vi "drive_straight4.vi"(4 "YawRate_Meas":dbl, 6 "YawTgt":dbl, 7 "Output Power Limit":dbl=0.35 format="%#_13g", 8 "YawMeas":dbl, 9 "Init":bool, 10 "DistanceTgt":dbl, 11 "EncoderVal":T1) -> (2 "Done":bool, 3 "MotorCmdOut":cluster{"left":dbl, "right":dbl})   [LabVIEW 2015]
panel:
  in  "Ernie DC_Yaw_Kp":dbl=0.03
  out "Drive":cluster{dbl, "Output Power Limit":dbl}(graph)
  out "DiffCtrl":cluster{dbl, "Output Power Limit":dbl}(graph)
  out "Yaw Graph":dbl(graph)
  in  "Position Error Limit Negative":dbl=-4.0
  in  "Position Error Limit Positive":dbl
  in  "DC_Yaw_Kd":dbl
  in  "DC_Yaw_Ki":dbl
  in  "Bert DC_Yaw_Kp":dbl=0.03
  in  "DC_NoYaw_Ki":dbl
  in  "DC_NoYaw_Kp":dbl
  in  "AC Rate Limit":dbl=0.05
  in  "AC_Ki":dbl
  in  "AC_Kp":dbl=0.1
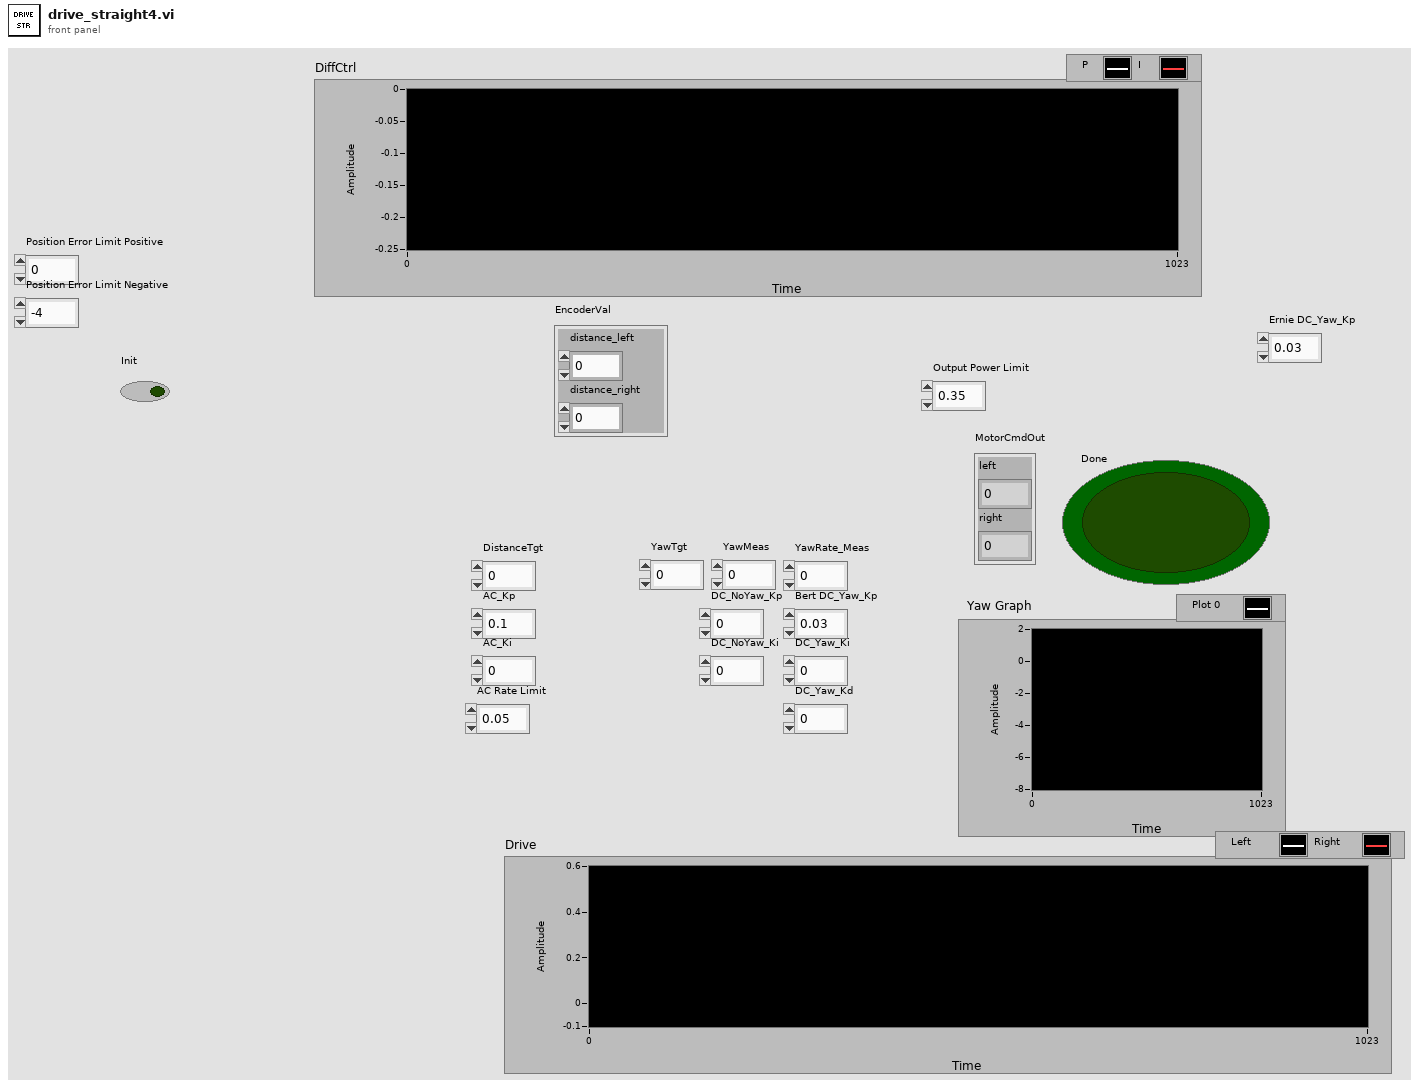
[diagram p1: front panel]
types:
  T1 = cluster{"distance_left":dbl, "distance_right":dbl}
  T2 = cluster{"Output Power Limit":dbl, "Output Power Limit":dbl}
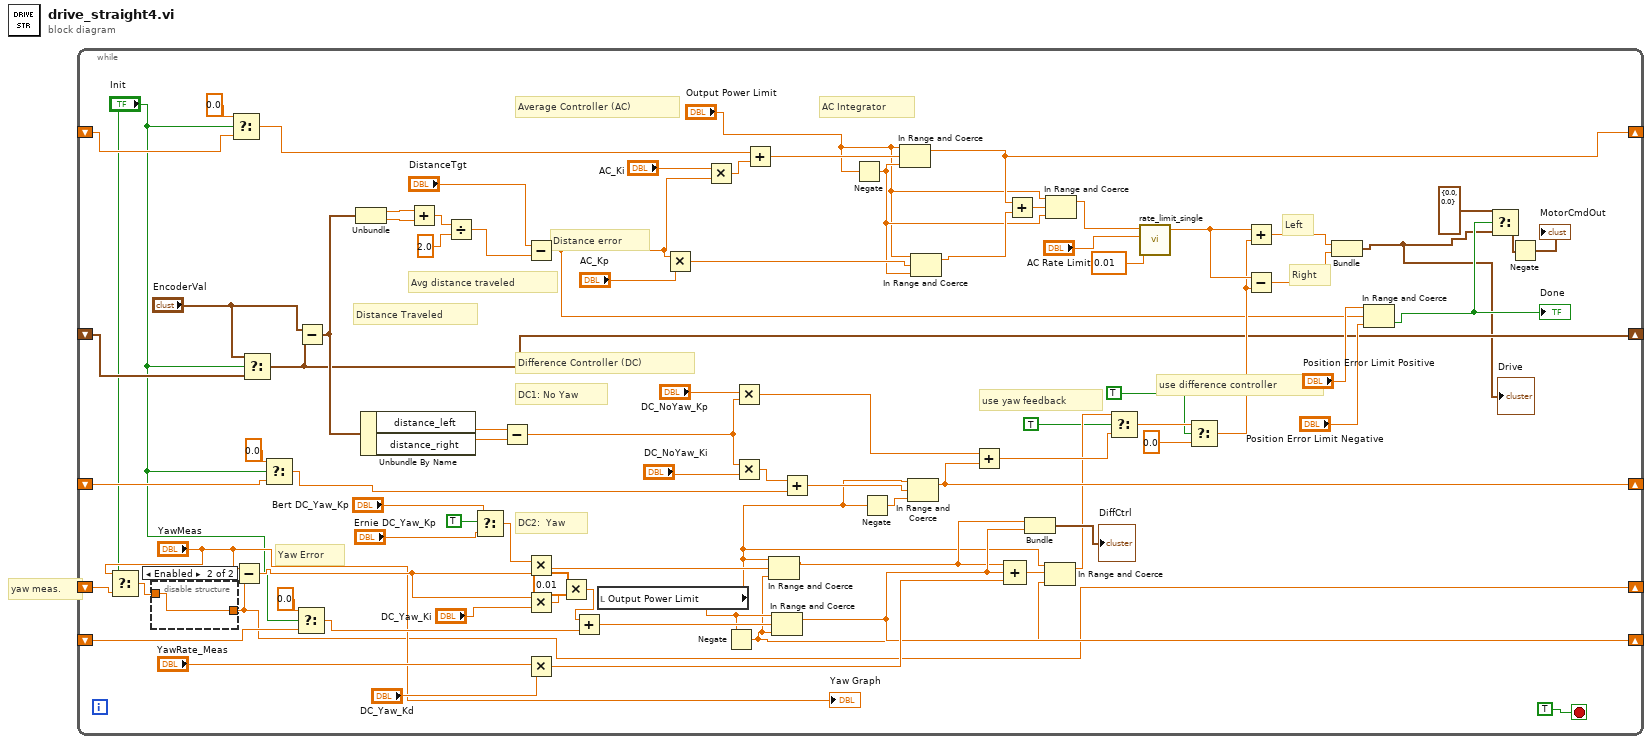
[diagram p0: block diagram]
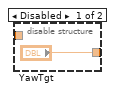
[diagram p2: hidden frame]
diagram:
  # "yaw meas."
  n1 = while {
    shift-right: [w34] -> _
    shift-left: _ -> [w33]
    shift-right: [w40] -> _
    shift-left: _ -> [w66]
    shift-right: [w37] -> _
    shift-left: _ -> [w62]
    shift-right: [w29] -> _
    shift-left: _ -> [w52]
    shift-right: [w7] -> _
    shift-left: _ -> [w6]
    stop <- TRUE stop-if-true
    # "use yaw feedback"
    # "use difference controller"
    # "Right"
    # "Left"
    # "Yaw Error"
    # "AC Integrator"
    # "Distance Traveled"
    # "Distance error"
    # "Avg distance traveled"
    # "DC2:  Yaw"
    # "DC1: No Yaw"
    # "Difference Controller (DC)"
    # "Average Controller (AC)"
    n2 = Select(t="YawMeas", s="Init", f=w6) -> (s? t:f=w9:dbl)
    n3 = disable-structure shown="Enabled" {
      disable-tunnel: ["YawTgt" w88] -> w7
      disable-tunnel: w9 -> [_ w88]
      frame Disabled {
      }
      frame Enabled {
      }
    }
    n4 = Select(t=0.0, s="Init", f=w66) -> (s? t:f=w65:dbl)
    n5 = Subtract(x="YawMeas", y=w7) -> (x-y=w55:dbl)
    n6 = Select(t="EncoderVal", s="Init", f=w33) -> (s? t:f=w34:T1)
    n7 = Select(t=0.0, s="Init", f=w62) -> (s? t:f=w61:dbl)
    n8 = Select(t=0.0, s="Init", f=w52) -> (s? t:f=w51:dbl)
    n9 = Subtract(x="EncoderVal", y=w34) -> (x-y=w73:T1)
    n10 = Unbundle(w73) -> ("distance_left"=w85:dbl, "distance_right"=w84:dbl)
    n11 = Unbundle By Name(w73) -> ("distance_left"=w72:dbl, "distance_right"=w71:dbl)
    n12 = Add(x=w85, y=w84) -> (x+y=w83:dbl)
    n13 = Divide(x=w83, y=2.0) -> (x/y=w25:dbl)
    n14 = Select(t="Bert DC_Yaw_Kp", s=TRUE, f="Ernie DC_Yaw_Kp") -> (s? t:f=w2:dbl)
    n15 = Subtract(x=w72, y=w71) -> (x-y=w69:dbl)
    n16 = Subtract(x="DistanceTgt", y=w25) -> (x-y=w44:dbl)
    n17 = Multiply(x=w2, y=w55) -> (x*y=w20:dbl)
    n18 = Multiply(x=w55, y="DC_Yaw_Ki") -> (x*y=w32:dbl)
    n19 = Multiply(x="YawRate_Meas", y="DC_Yaw_Kd") -> (x*y=w54:dbl)
    n20 = Multiply(x=0.01, y=w32) -> (x*y=w31:dbl)
    n21 = Add(x=w31, y=w51) -> (x+y=w39:dbl)
    n22 = local read "Output Power Limit"() -> (w16:dbl)
    n23 = Multiply(x=w44, y="AC_Kp") -> (x*y=w27:dbl)
    n24 = Multiply(x="AC_Ki", y=w44) -> (x*y=w80:dbl)
    n25 = Negate(x=w16) -> (-x=w15:dbl)
    n26 = Multiply(x="DC_NoYaw_Kp", y=w69) -> (x*y=w60:dbl)
    n27 = Multiply(x=w69, y="DC_NoYaw_Ki") -> (x*y=w67:dbl)
    n28 = Add(x=w65, y=w80) -> (x+y=w41:dbl)
    n29 = In Range and Coerce(upper limit=w16, x=w20, lower limit=w15) -> (coerced(x)=w19:dbl)  [unwired: 1 out]
    n30 = In Range and Coerce(upper limit=w16, x=w39, lower limit=w15) -> (coerced(x)=w29:dbl)  [unwired: 1 out]
    n31 = Add(x=w67, y=w61) -> (x+y=w36:dbl)
    n32 = Negate(x="Output Power Limit") -> (-x=w21:dbl)
    n33 = Negate(x=w16) -> (-x=w38:dbl)
    n34 = In Range and Coerce(upper limit="Output Power Limit", x=w41, lower limit=w21) -> (coerced(x)=w40:dbl)  [unwired: 1 out]
    n35 = In Range and Coerce(upper limit=w16, x=w36, lower limit=w38) -> (coerced(x)=w37:dbl)  [unwired: 1 out]
    n36 = In Range and Coerce(upper limit="Output Power Limit", x=w27, lower limit=w21) -> (coerced(x)=w26:dbl)  [unwired: 1 out]
    n37 = Add(x=w60, y=w37) -> (x+y=w59:dbl)
    n38 = Compound Arithmetic op=ADD(w19, w29, w54) -> (w18:dbl)
    n39 = Add(x=w40, y=w26) -> (x+y=w23:dbl)
    n40 = Bundle("Output Power Limit"=w19, "Output Power Limit"=w29) -> (→"DiffCtrl":T2)  [unwired: 1 in]
    n41 = In Range and Coerce(upper limit=w16, x=w18, lower limit=w15) -> (coerced(x)=w17:dbl)  [unwired: 1 out]
    n42 = In Range and Coerce(upper limit="Output Power Limit", x=w23, lower limit=w21) -> (coerced(x)=w22:dbl)  [unwired: 1 out]
    n43 = Select(t=w17, s=TRUE ("Use Yaw Feedback?"), f=w59) -> (s? t:f=w49:dbl)
    n44 = call "rate_limit_single.vi"("Sample Period"=0.01, "Rate Limit"="AC Rate Limit", "Input"=w22) -> ("Output"=w76:dbl)  [unwired: 8 in]
    n45 = Select(t=w49, s=TRUE ("Enable Difference Controller"), f=0.0) -> (s? t:f=w50:dbl)
    n46 = Add(x=w76, y=w50) -> (x+y=w75:dbl)
    n47 = Subtract(x=w76, y=w50) -> (x-y=w74:dbl)
    n48 = Bundle(w75, w74) -> (w13:cluster{dbl, dbl})  [unwired: 1 in]
    "Drive" <- w13
    n49 = In Range and Coerce(upper limit="Position Error Limit Positive", x=w44, lower limit="Position Error Limit Negative") -> (In Range?=w43:bool)  [unwired: 1 out]
    "Done" <- w43
    n50 = Select(t=T2 {"Output Power Limit"=0.0, "Output Power Limit"=0.0}, s=w43, f=w13) -> (s? t:f=w11:T2)
    n51 = Negate(x=w11) -> (-x=→"MotorCmdOut":T2)
    "Yaw Graph" <- "YawMeas"
  }
